vi "Drink.vi"(8 "Error In":errorcluster, 11 "reference in":refnum<class "OolingMilkTea.lvclass">) -> (0 "Error Out":errorcluster, 3 "reference out":refnum<class "OolingMilkTea.lvclass">)   [LabVIEW 2020, in "OolingMilkTea.lvclass"]
uses:
  OolingMilkTea.lvclass
  Console_class/Console.lvclass
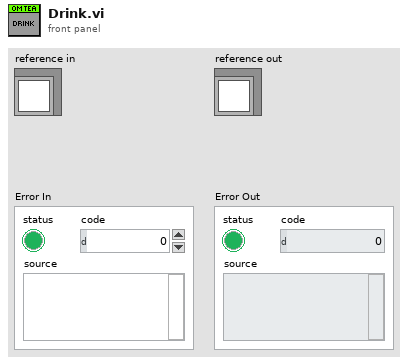
[diagram p1: front panel]
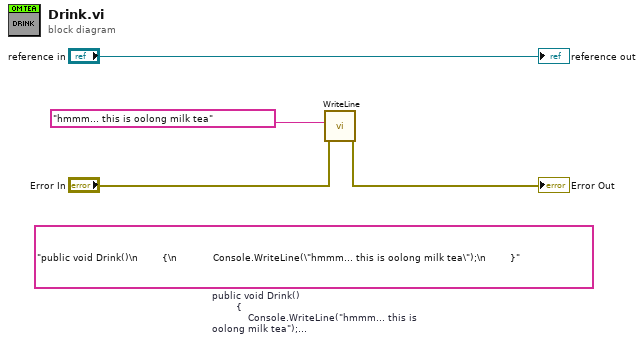
[diagram p0: block diagram]
diagram:
  (unwired) "public void Drink()\n        {\n            Console.WriteLine(\"hmmm... this is oolong milk tea\");\n        }"  # public void Drink()         {             Console.WriteLine("hmmm... this is oolong milk tea");         }
  n1 = call "WriteLine.vi"("Error In"="Error In", "ConsoleText"="hmmm... this is oolong milk tea") -> ("Error Out"=→"Error Out":errorcluster)  [unwired: 9 in]
  "reference out" <- "reference in"
